vi "Write MCCW ACLR Config.vi"(10 "MCCW ACLR Config":T1 {"Carriers"."Array" format="%#_6p"; "Power"."Array" format="%#_6p"; "Frequency"."Array" format="%#_6p"}, 11 "MCCW ACLR in":refnum<class "MCCW ACLR.lvclass">) -> (3 "MCCW ACLR out":refnum<class "MCCW ACLR.lvclass">)   [LabVIEW 2020, in "MCCW ACLR.lvclass"]
uses:
  MCCW ACLR.lvclass
  Controls/ACLR configuration.ctl
  MCCW ACLR.lvclass/MCCW ACLR.ctl
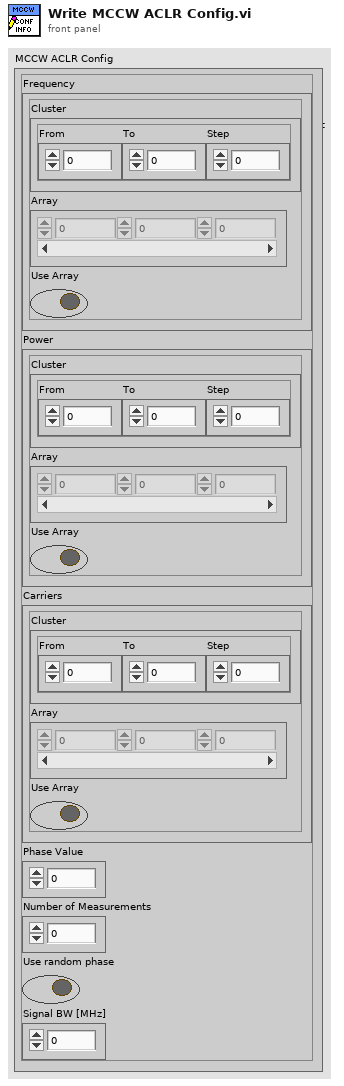
[diagram p1: front panel]
types:
  T1 = typedef "MCCW ACLR.lvclass/ACLR configuration.ctl" = cluster{"Frequency":cluster{"Cluster ":cluster{"From":dbl, "To":dbl, "Step":dbl}, "Array":dbl[], "Use Array":bool}, "Power":cluster{"Cluster ":cluster{"From":dbl, "To":dbl, "Step":dbl}, "Array":dbl[], "Use Array":bool}, "Carriers":cluster{"Cluster ":cluster{"From":dbl, "To":dbl, "Step":dbl}, "Array":dbl[], "Use Array":bool}, "Phase Value":dbl, "Number of Measurements":u32, "Use random phase":bool, "Signal BW [MHz] ":dbl}
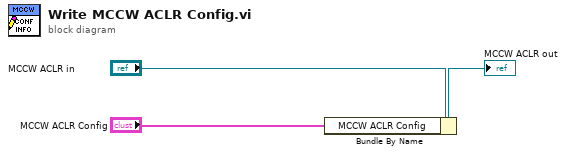
[diagram p0: block diagram]
diagram:
  n1 = Bundle By Name(cluster="MCCW ACLR in", "MCCW ACLR Config"="MCCW ACLR Config") -> (→"MCCW ACLR out":refnum<class "MCCW ACLR.lvclass">)
